vi "bindQueueToExchange.vi"(0 "RabbitMQ Session In":T1, 5 "Exchange Name In":string, 7 "Queue Name In":string, 9 "Routing Key In":string, 11 "error in (no error)":errorcluster) -> (4 "RabbitMQ Session Out":T1, 6 "Exchange Name out":string, 8 "Queue Name out":string, 10 "Routing Key out":string, 15 "error out":errorcluster)   [LabVIEW 2019, in "rabbitmq.lvlib"]
uses:
  rabbitmq.lvlib
  session.ctl
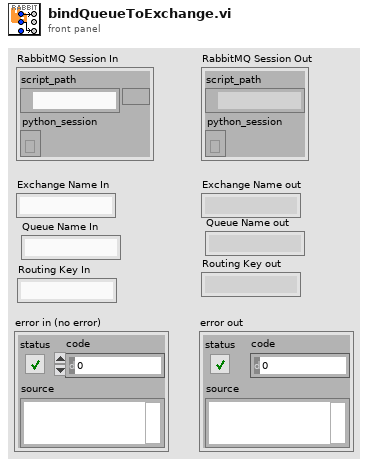
[diagram p1: front panel]
types:
  T1 = typedef "rabbitmq.lvlib/session.ctl" = cluster{"script_path":path, "python_session":refnum<k35>}
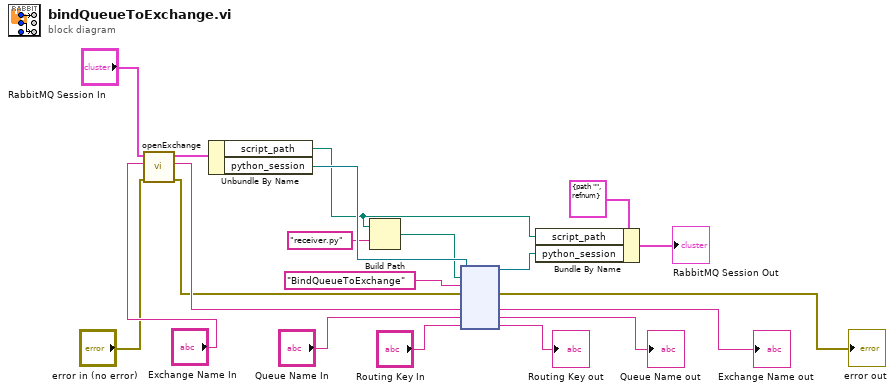
[diagram p0: block diagram]
diagram:
  n1 = call "openExchange.vi"("error in (no error)"="error in (no error)", "Exchange Name In"="Exchange Name In", "RabbitMQ Session In"="RabbitMQ Session In") -> ("error out"=w1:errorcluster, "Exchange Name out"=w3:string, "RabbitMQ Session Out"=w5:T1)  [unwired: 6 in]
  n2 = Unbundle By Name(w5) -> ("script_path"=w13:path, "python_session"=w16:refnum<k35>)
  n3 = Build Path(base path=w13, name or relative path="receiver.py") -> (appended path=w12:path)
  n4 = node(w16, w12, "BindQueueToExchange" ("function name"), w1, w3, "Queue Name In", "Routing Key In") -> (w19:refnum<k35>, →"error out":errorcluster, →"Exchange Name out":string, →"Queue Name out":string, →"Routing Key out":string)  [unwired: 2 in, 2 out]
  n5 = Bundle By Name(cluster=T1 {"script_path"=path "", "python_session"=refnum}, "script_path"=w13, "python_session"=w19) -> (→"RabbitMQ Session Out":T1)
